vi "ATE_BSE-Event_Enqueue.vi"(8 "error in (no error)":errorcluster, 11 "Event":T1) -> (0 "error out":errorcluster)   [LabVIEW 2021]
uses:
  Controls/ATE_BSE_Event_type_def.ctl
  Controls/ATE_BSE_Queue_Operations.ctl
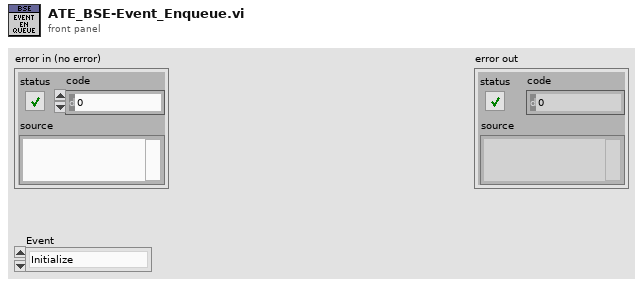
[diagram p1: front panel]
types:
  T1 = typedef "ATE_BSE_Event_type_def.ctl" = enum16{"Initialize", "Configure", "Ip Simulation", "IMS", "ECall", "Exit", "Error"}
  T2 = typedef "ATE_BSE_Queue_Operations.ctl" = enum16{"Init", "Get Queue", "Flush", "Close"}
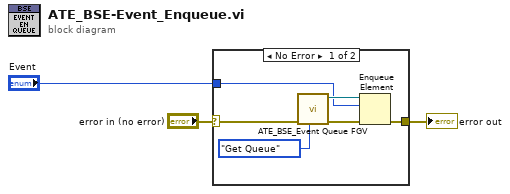
[diagram p0: block diagram]
diagram:
  n1 = case shown="No Error" "error in (no error)" {
    selector: "error in (no error)" -> [w9 w10]
    tunnel: [w7 w10] -> w3
    tunnel: "Event" -> [w4 _]
    frame No Error {
      n2 = call "ATE_BSE_Event Queue FGV.vi"("Operations"=ATE_BSE_Queue_Operations."Get Queue", "error in (no error)"=w9) -> ("error out"=w8:errorcluster, "queue out"=w5:refnum<queue>)  [unwired: 8 in]
      n3 = Enqueue Element(queue=w5, element=w4, error in (no error)=w8) -> (error out=w7:errorcluster)  [unwired: 1 in, 2 out]
    }
    frame Error {
    }
  }
  "error out" <- w3
